vi "CRYMessage Set DigitalIO Ports.vi"(6 "RawPort 2 Pattern":u8 format="%x", 9 "Port 2 Pattern":u8 format="%x", 11 "Port 1 Pattern":u8 format="%x") -> (1 "Pattern2 Result":bool, 2 "bInited":bool, 3 "Pattern1 Result":bool)   [LabVIEW 2013]
uses:
  CRYMessage Global.vi
  Hardware/SubVI/CRY6175APT_Win32.dll
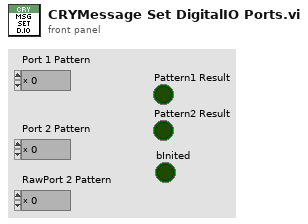
[diagram p1: front panel]
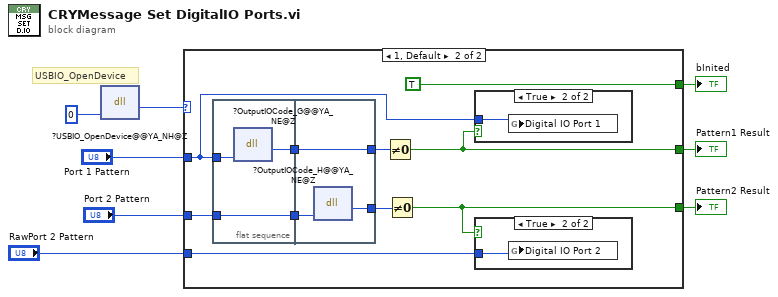
[diagram p0: block diagram]
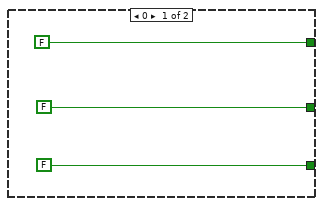
[diagram p2: hidden frame]
diagram:
  # "USBIO_OpenDevice"
  n1 = dll-call lib="I:/Work/CRY6181/CRYSystem/Hardware/SubVI/CRY6175APT_Win32.dll" fn="?USBIO_OpenDevice@@YA_NH@Z"("nDevID"=0) -> ("return type"=w7:i32)  [unwired: 4 in, 2 out]
  n2 = case shown="1, Default" w7 {
    tunnel: "Port 1 Pattern" -> [_ w12]
    tunnel: "Port 2 Pattern" -> [_ w15]
    tunnel: [FALSE w16] -> w4
    tunnel: [FALSE w14] -> w3
    tunnel: [FALSE TRUE] -> w2
    tunnel: "RawPort 2 Pattern" -> [_ w13]
    frame 0 {
    }
    frame 1, Default {
      n3 = flat-sequence {
        tunnel: w12 -> [w26]
        tunnel: w15 -> [w25]
        tunnel: [w25] -> w21
        tunnel: [w24] -> w20
        tunnel: w21 -> [w29]
        tunnel: [w28] -> w19
        tunnel: w20 -> [w28]
        tunnel: [w27] -> w18
        frame #0 {
          n4 = dll-call lib="I:/Work/CRY6181/CRYSystem/Hardware/SubVI/CRY6175APT_Win32.dll" fn="?OutputIOCode_G@@YA_NE@Z"("Pattern"=w26) -> ("return type"=w24:i32)  [unwired: 4 in, 2 out]
        }
        frame #1 {
          n5 = dll-call lib="I:/Work/CRY6181/CRYSystem/Hardware/SubVI/CRY6175APT_Win32.dll" fn="?OutputIOCode_H@@YA_NE@Z"("Pattern"=w29) -> ("return type"=w27:i32)  [unwired: 4 in, 2 out]
        }
      }
      n6 = Not Equal To 0?(x=w19) -> (x != 0?=w16:bool)
      n7 = Not Equal To 0?(x=w18) -> (x != 0?=w14:bool)
      n8 = case shown="True" w16 {
        tunnel: w12 -> [_ w23]
        frame False {
        }
        frame True {
          n9 = global write "CRYMessage Global.vi" "Digital IO Port 1"(w23) -> ()
        }
      }
      n10 = case shown="True" w14 {
        tunnel: w13 -> [_ w22]
        frame False {
        }
        frame True {
          n11 = global write "CRYMessage Global.vi" "Digital IO Port 2"(w22) -> ()
        }
      }
    }
  }
  "Pattern1 Result" <- w4
  "Pattern2 Result" <- w3
  "bInited" <- w2
